vi "registration-test.vi"(8 "error in (no error)":errorcluster) -> (0 "error out":errorcluster)   [LabVIEW 2013]
uses:
  src/SMO/SMO.lvclass
  <vilib>/addons/_JKI Toolkits/Caraya/classes/Test/Test.lvclass
  src/Registry/Registry-SMO.lvclass
  <vilib>/addons/_JKI Toolkits/Caraya/classes/Assert/Assert.lvclass
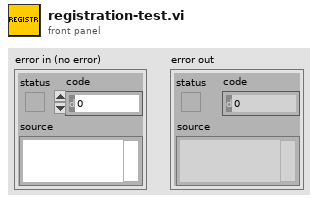
[diagram p1: front panel]
types:
  T1 = typedef "Registry-SMO.lvclass/PublicRegistryEvents--Cluster.ctl" = cluster{"Register Event":refnum<user-event>, "Unregister Event":refnum<user-event>}
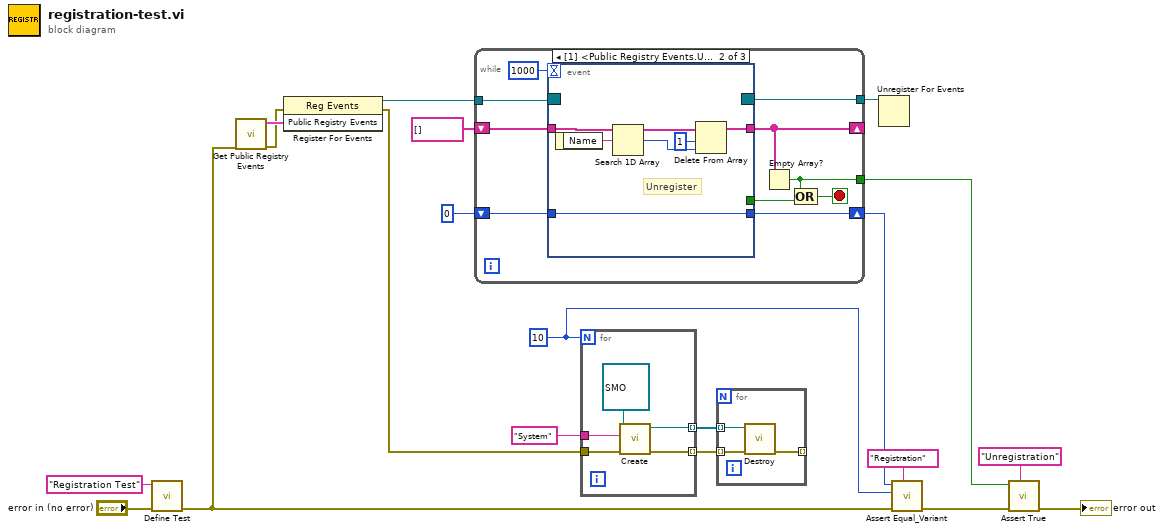
[diagram p0: block diagram]
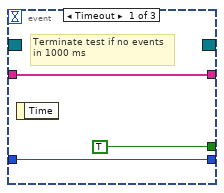
[diagram p2: hidden frame]
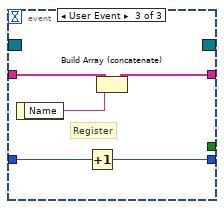
[diagram p3: hidden frame]
diagram:
  w5 = 10
  n1 = call <vilib>:"Define Test.vi"("error in (no error)"="error in (no error)", "Label (VI Title)"="Registration Test") -> ("error out"=w8:errorcluster)  [unwired: 9 in]
  n2 = call "Get Public Registry Events.vi"("error in (no error)"=w8) -> ("error out"=w9:errorcluster, "Public Registry Events"=w17:T1)  [unwired: 9 in]
  n3 = register-events(error in=w9, w17) -> (reference out=w16:refnum<event-registration>, error out=w10:errorcluster)  [unwired: 1 in]
  n4 = while {
    tunnel: w16 -> [w30]
    shift-right: [w28] -> _
    shift-left: string[] [] -> [w29]
    tunnel: [w27] -> w14
    shift-right: [w26] -> w6
    shift-left: 0 -> [w25]
    tunnel: [w21] -> w2
    stop <- w22 stop-if-true
    n5 = event shown="[1] <Public Registry Events.Unregister Event>: User Event" {
      selector: w30 -> [_ _ _]
      dyn-events: [_ _ _] -> w27
      timeout: 1000 -> [_ _ _]
      tunnel: w29 -> [w33 w38 w44]
      tunnel: [w33 w37 w42] -> w28
      tunnel: [w32 w34 w41] -> w26
      tunnel: w25 -> [w32 w34 w40]
      tunnel: [TRUE _ _] -> w23
      event Timeout {
        # "Terminate test if no events\nin 1000 ms"
        n6 = event-data() -> ()  [unwired: 1 in, 1 out]
      }
      event User Event {
        # "Unregister"
        n7 = event-data() -> ("Name"=w39:string)  [unwired: 1 in]
        n8 = Search 1D Array(1D array=w38, element=w39) -> (index of element=w36:i32)  [unwired: 1 in]
        n9 = Delete From Array(array=w38, length=1, index=w36) -> (array with subset deleted=w37:string[])  [unwired: 1 out]
      }
      event User Event {
        # "Register"
        n10 = event-data() -> ("Name"=w43:string)  [unwired: 1 in]
        n11 = Increment(x=w40) -> (x+1=w41:i32)
        n12 = Build Array (concatenate)(w44, w43) -> (w42:string[])
      }
    }
    n13 = Empty Array?(array=w28) -> (empty?=w21:bool)
    n14 = Compound Arithmetic op=OR(w21, w23) -> (w22:bool)
  }
  n15 = for {
    N: w5 -> [_]
    tunnel: "System" ("Subsystem Name (optional)") -> [w48]
    tunnel: [w47] -> w12 mode=indexing
    tunnel: [w46] -> w11 mode=indexing
    tunnel: w10 -> [w45]
    n16 = call "Create.vi"("error in (no error)"=w45, "Subsystem Name (optional)"=w48, "SMO"=refnum<class "SMO.lvclass"> refnum ("SMO.lvclass")) -> ("error out"=w46:errorcluster, "SMO out"=w47:refnum<class "SMO.lvclass">)  [unwired: 6 in, 1 out]
  }
  n17 = for {
    tunnel: w12 -> [w52] mode=indexing
    tunnel: [w51] -> _ mode=indexing
    tunnel: w11 -> [w50] mode=indexing
    n18 = call "Destroy.vi"("error in (no error)"=w50, "SMO"=w52) -> ("error out"=w51:errorcluster)  [unwired: 9 in]
  }
  n19 = Unregister For Events(event registration refnum=w14) -> ()  [unwired: 1 in, 1 out]
  n20 = call <vilib>:"Assert Equal_Variant.vi"("Label"="Registration" ("Label (VI Title)"), "error in (no error)"=w8, "Y"=w5, "X"=w6) -> ("error out"=w4:errorcluster)  [unwired: 7 in]
  n21 = call <vilib>:"Assert True.vi"("Label"="Unregistration" ("Label (VI Title)"), "error in (no error)"=w4, "True?"=w2) -> ("error out"=→"error out":errorcluster)  [unwired: 8 in]
